vi "C-Scan (LLC messages).vi"(7 "Micropulse # In":i32, 8 "Define C-Scan Index":T1={"Index Start"=0.0, "Index Length"=260.0, "Indexing\nResolution"=5.0, "Ch1 Start"=0.0, "Ch1 Finish"=0.0, "Ch2 Start"=0.0, "Ch2 Finish"=0.0} {"Ch2 Finish" format="%#_6f"; "Ch2 Start" format="%#_6f"; "Ch1 Finish" format="%#_6f"; "Ch1 Start" format="%#_6f"; "Index Start" format="%#_6f"; "Index Length" format="%#_6f"; "Indexing\nResolution" format="%#_6f"}, 9 "Scan definition":T2={"Scan Start"=0.0, "Scan Length"=280.0, "Inspection Resolution"=0.5, "Direction"=enum."Forwards"} {"Inspection Resolution" format="%#_6f"; "Scan Start" format="%#_6f"; "Scan Length" format="%#_6f"}, 10 "Axis No.":u8=1 min=1 max=4, 11 "scan data info":T4 {"Error Message" format="%04x"; "Message Header" format="%04x"; "IP"."MIP location" format="%#.0f"; "IP"."Location" format="%#.0f"; "PRF" format="%.0fHz"}) -> (0 "Update Display?":bool, 1 "C-Scan In Progress?":bool, 2 "B-Scan index":i32, 3 "C-Scan Out":u16[][](array[numeric]))   [LabVIEW 2026, in "MicroPulse_Driver.lvlib"]
uses:
  MicroPulse_Driver.lvlib
  Data/Datatypes/MP - scan data info.ctl
  Data/Datatypes/MP - data output format.ctl
  Data/Datatypes/MP - retain scan.ctl
  Data/Datatypes/MP - axis positions (LLC).ctl
  Data/Datatypes/MP - fly scan range.ctl
  Data/Datatypes/MP - inspection direction.ctl
  Data/Datatypes/MP - C-Scan Definition.ctl
  Low Level/FGV - C-Scan Active - Action [Enum].ctl
  <instrlib>/Micropulse/Micropulse.lvlib
panel:
  out "C-Scan index":i32
  # "C-Scan Index"
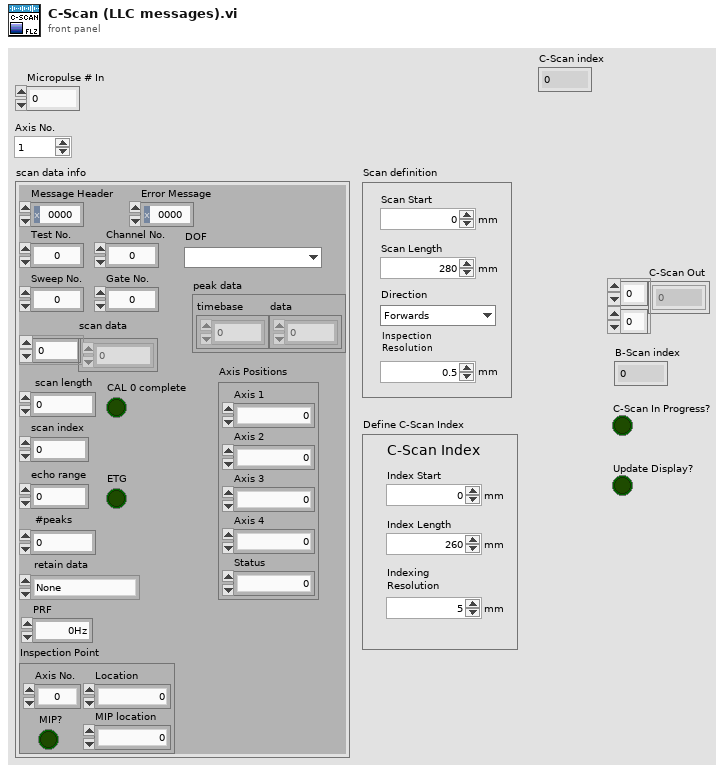
[diagram p1: front panel]
types:
  T1 = typedef "Micropulse.lvlib/MP - C-Scan Definition.ctl" = cluster{"Index Start":dbl, "Index Length":dbl, "Indexing\nResolution":dbl, "Ch1 Start":dbl, "Ch1 Finish":dbl, "Ch2 Start":dbl, "Ch2 Finish":dbl}
  T2 = typedef "Micropulse.lvlib/MP - fly scan range.ctl" = cluster{"Scan Start":dbl, "Scan Length":dbl, "Inspection Resolution":dbl, "Direction":T3}
  T3 = typedef "Micropulse.lvlib/MP - inspection direction.ctl" = enum16{"Forwards", "Backwards"}
  T4 = typedef "Micropulse.lvlib/MP - scan data info.ctl" = cluster{"Message Header":u16, "Error Message":u16, "Test No.":u32, "Channel No.":u8, "Sweep No.":u32, "Gate No.":u32, "DOF":T5, "retain data":T6, "scan data":u16[], "scan length":i32, "scan index":i32, "peak data":cluster{"timebase":u16[], "data":u16[]}, "#peaks":i32, "PRF":dbl, "IP":cluster{"Axis No.":u8, "Location":u32, "MIP location":u32, "MIP?":bool}, "echo range":u16, "ETG":bool, "CAL 0 complete":bool, "Axis Positions":T7}
  T5 = typedef "Micropulse.lvlib/MP - data output format.ctl" = enum16{"", "8-bit Mode", "10-bit Mode", "12-bit Mode", "16-bit Mode", "8-bit Log Mode", "12-bit Packed Mode"}
  T6 = typedef "Micropulse.lvlib/MP - retain scan.ctl" = enum16{"None", "Ascan", "Peaks"}
  T7 = typedef "Micropulse.lvlib/MP - axis positions (LLC).ctl" = cluster{"Axis 1":u32, "Axis 2":u32, "Axis 3":u32, "Axis 4":u32, "Status":u8}
  T8 = typedef "MicroPulse_Driver.lvlib/FGV - C-Scan Active - Action [Enum].ctl" = enum16{"Read", "Read & Reset Start Flag", "Start C-Scan", "C-Scan Finished"}
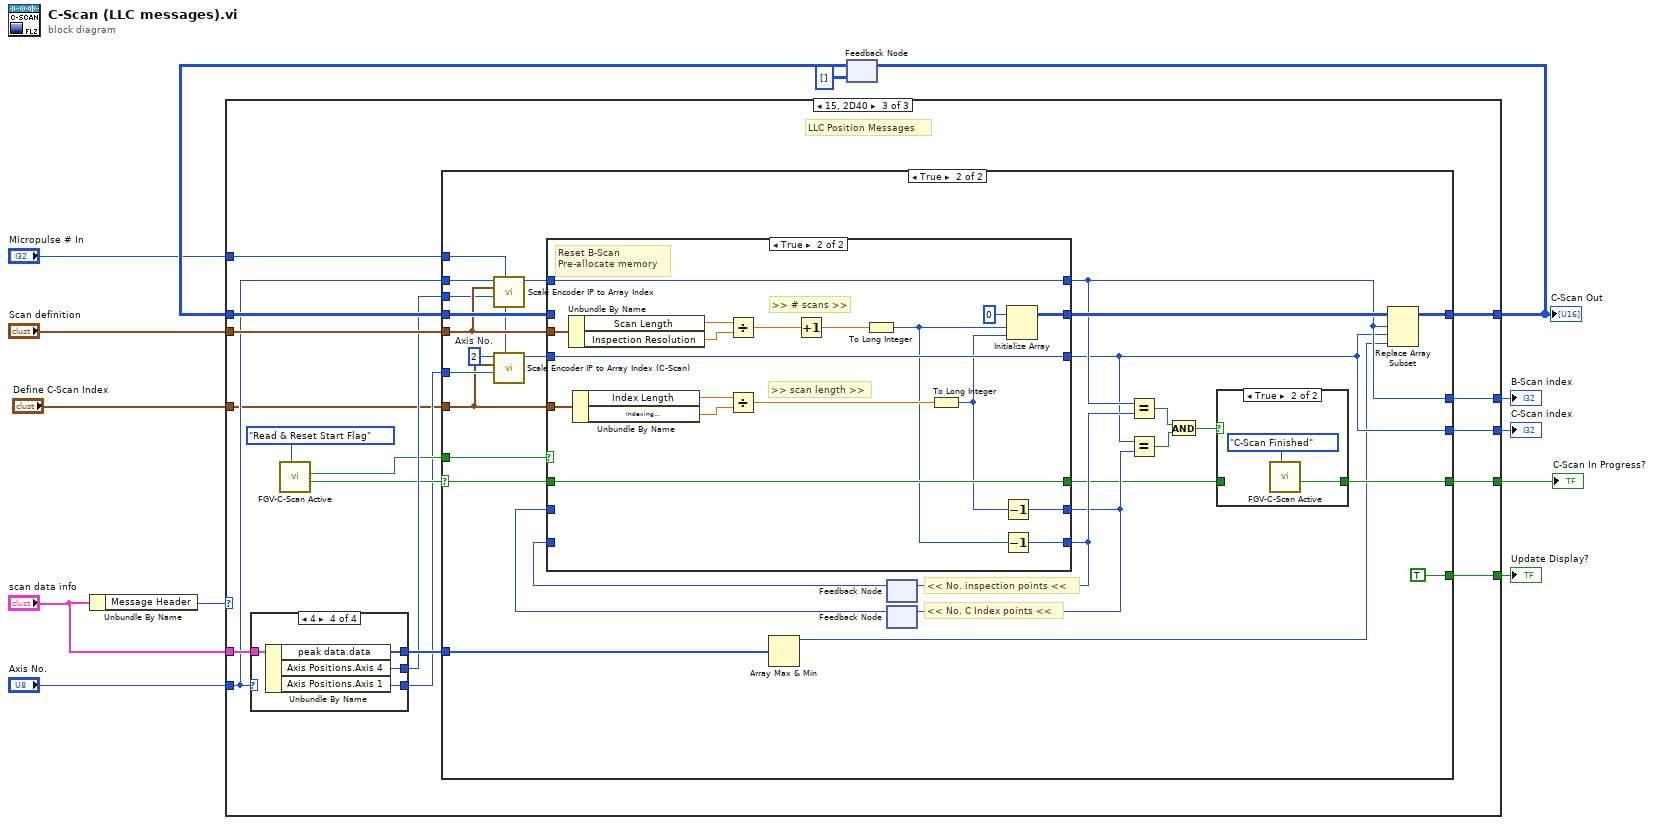
[diagram p0: block diagram]
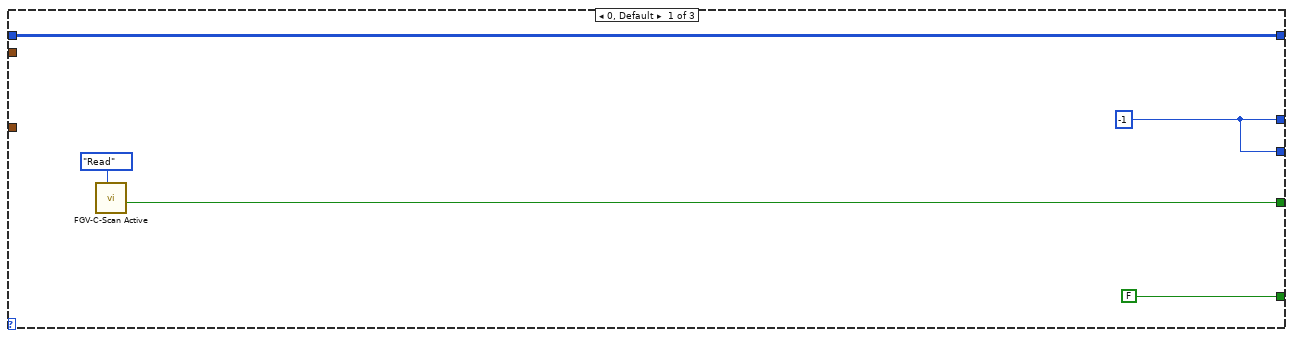
[diagram p2: hidden frame]
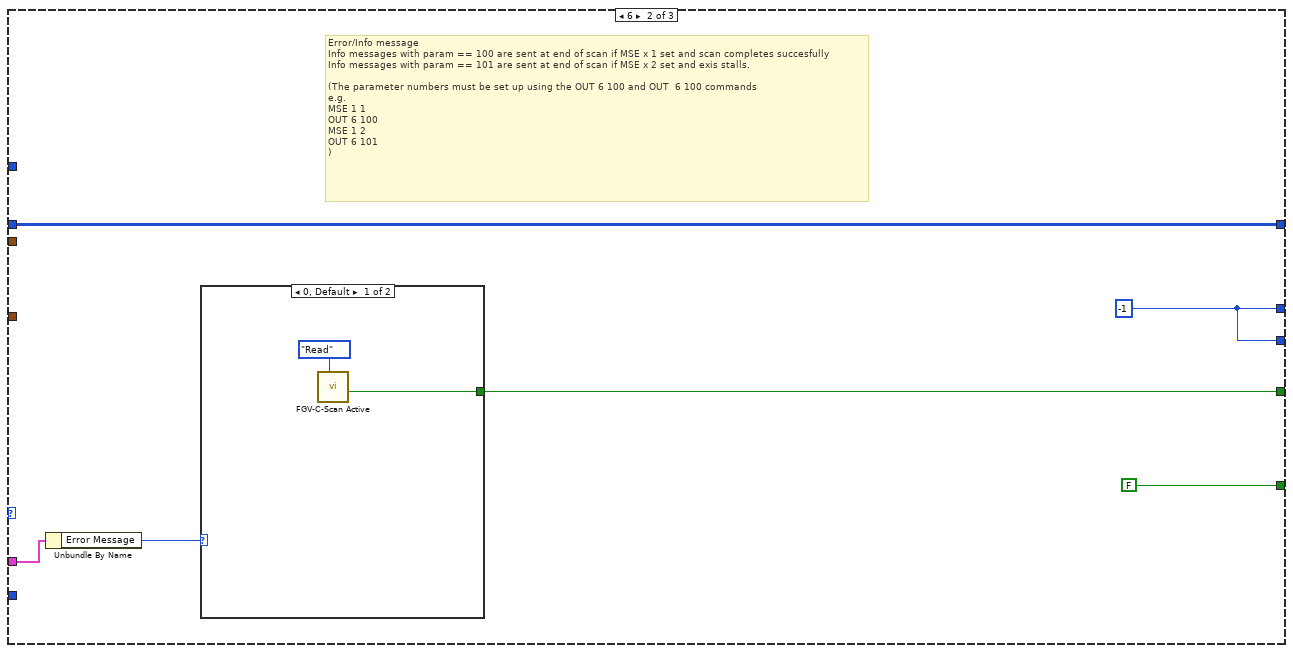
[diagram p3: hidden frame]
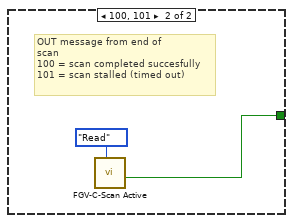
[diagram p4: hidden frame]
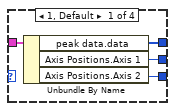
[diagram p5: hidden frame]
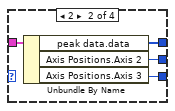
[diagram p6: hidden frame]
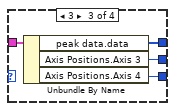
[diagram p7: hidden frame]
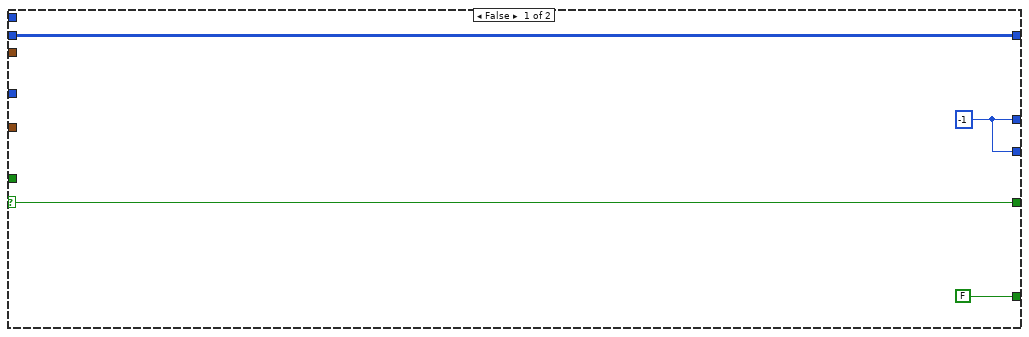
[diagram p8: hidden frame]
diagram:
  n1 = Unbundle By Name("scan data info") -> ("Message Header"=w13:u16)
  n2 = feedback #1(u16[][] []) -> (w9:u16[][])
  n3 = case shown="15, 2D40" w13 {
    tunnel: "scan data info" -> [_ w22 w45]
    tunnel: "Scan definition" -> [_ _ w39]
    tunnel: [w18 w24 w43] -> w10
    tunnel: w9 -> [w18 w24 w42]
    tunnel: "Micropulse # In" -> [_ _ w38]
    tunnel: [w14 w20 w41] -> w6
    tunnel: [FALSE FALSE w40] -> w5
    tunnel: "Axis No." -> [_ _ w36]
    tunnel: [w16 w19 w35] -> w3
    tunnel: "Define C-Scan Index" -> [_ _ w30]
    tunnel: [w16 w19 w29] -> w1
    frame 0, Default {
      w16 = -1 ("B-Scan index")
      n4 = call "FGV-C-Scan Active.vi"("Action"=FGV_-_C-Scan_Active_-_Action_[Enum]."Read") -> ("C-Scan In Progress?"=w14:bool)  [unwired: 8 in, 2 out]
    }
    frame 6 {
      w19 = -1 ("B-Scan index")
      # "Error/Info message\nInfo messages with param == 100 are sent at end of scan if MSE x 1 set and scan completes succesfully\nInfo messages with param == 101 are sent at end of scan if MSE x 2 set and exis stalls.\n\n(The parameter numbers must be set up using the OUT 6 100 and OUT  6 100 commands \ne.g.\nMSE 1 1\nOUT 6 100\nMSE 1 2\nOUT 6 101\n)"
      n5 = Unbundle By Name(w22) -> ("Error Message"=w21:u16)
      n6 = case shown="0, Default" w21 {
        tunnel: [w25 w27] -> w20
        frame 0, Default {
          n7 = call "FGV-C-Scan Active.vi"("Action"=FGV_-_C-Scan_Active_-_Action_[Enum]."Read") -> ("C-Scan In Progress?"=w25:bool)  [unwired: 8 in, 2 out]
        }
        frame 100, 101 {
          # "OUT message from end of\nscan\n100 = scan completed succesfully\n101 = scan stalled (timed out)"
          n8 = call "FGV-C-Scan Active.vi"("Action"=FGV_-_C-Scan_Active_-_Action_[Enum]."Read") -> ("C-Scan In Progress?"=w27:bool)  [unwired: 8 in, 2 out]
        }
      }
    }
    frame 21, 11584 {
      # "LLC Position Messages"
      n9 = case shown="4" w36 {
        tunnel: w45 -> [w49 w53 w57 w61]
        tunnel: [w48 w52 w56 w60] -> w44
        tunnel: [w47 w51 w55 w59] -> w37
        tunnel: [w46 w50 w54 w58] -> w31
        frame 1, Default {
          n10 = Unbundle By Name(w49) -> ("peak data.data"=w48:u16[], "Axis Positions.Axis 1"=w47:u32, "Axis Positions.Axis 2"=w46:u32)
        }
        frame 2 {
          n11 = Unbundle By Name(w53) -> ("peak data.data"=w52:u16[], "Axis Positions.Axis 2"=w51:u32, "Axis Positions.Axis 3"=w50:u32)
        }
        frame 3 {
          n12 = Unbundle By Name(w57) -> ("peak data.data"=w56:u16[], "Axis Positions.Axis 3"=w55:u32, "Axis Positions.Axis 4"=w54:u32)
        }
        frame 4 {
          n13 = Unbundle By Name(w61) -> ("peak data.data"=w60:u16[], "Axis Positions.Axis 4"=w59:u32, "Axis Positions.Axis 1"=w58:u32)
        }
      }
      n14 = call "FGV-C-Scan Active.vi"("Action"=FGV_-_C-Scan_Active_-_Action_[Enum]."Read & Reset Start Flag") -> ("C-Scan In Progress?"=w33:bool, "C-Scan Start?"=w34:bool)  [unwired: 8 in, 1 out]
      n15 = case shown="True" w33 {
        selector: w33 -> [w64 w89]
        tunnel: w42 -> [w65 w93]
        tunnel: [w65 w91] -> w43
        tunnel: w44 -> [_ w86]
        tunnel: w39 -> [_ w84]
        tunnel: [w64 w68] -> w41
        tunnel: [FALSE TRUE] -> w40
        tunnel: w38 -> [_ w67]
        tunnel: w34 -> [_ w85]
        tunnel: w37 -> [_ w83]
        tunnel: w36 -> [_ w82]
        tunnel: [w62 w76] -> w35
        tunnel: w31 -> [_ w81]
        tunnel: w30 -> [_ w79]
        tunnel: [w62 w74] -> w29
        frame False {
          w62 = -1 ("B-Scan index")
        }
        frame True {
          w80 = u8 2  # Axis No.
          # "<< No. C Index points <<"
          # "<< No. inspection points <<"
          n16 = call "Scale Encoder IP to Array Index.vi"("Micropulse # In"=w67, "Inspection Point Location"=w83, "Scan definition"=w84, "Axis No."=w82) -> ("B-Scan index"=w87:i32)  [unwired: 6 in, 1 out]
          n17 = call "Scale Encoder IP to Array Index (C-Scan).vi"("Micropulse # In"=w67, "Inspection Point Location"=w81, "Define C-Scan Index"=w79, "Axis No."=w80) -> ("C-Scan index"=w78:i32)  [unwired: 6 in, 1 out]
          n18 = Array Max & Min(array=w86) -> (max value=w66:u16)  [unwired: 3 out]
          n19 = feedback #2() -> (w90:i32)  [unwired: 1 in]
          n20 = feedback #3() -> (w77:i32)  [unwired: 1 in]
          n21 = case shown="True" w85 {
            tunnel: w93 -> [w102 _]
            tunnel: [w102 w120] -> w92
            tunnel: w84 -> [_ w118]
            tunnel: w87 -> [w100 w112]
            tunnel: [w99 w115] -> w75
            tunnel: w90 -> [w99 _]
            tunnel: [w101 w113] -> w69
            tunnel: w89 -> [w101 w113]
            tunnel: [w100 w112] -> w76
            tunnel: w79 -> [_ w109]
            tunnel: [w98 w108] -> w74
            tunnel: w78 -> [w98 w108]
            tunnel: [w97 w106] -> w73
            tunnel: w77 -> [w97 _]
            frame False {
            }
            frame True {
              # "Reset B-Scan\nPre-allocate memory"
              # ">> scan length >>"
              # ">> # scans >>"
              n22 = Unbundle By Name(w118) -> ("Scan Length"=w117:dbl, "Inspection Resolution"=w116:dbl)
              n23 = Unbundle By Name(w109) -> ("Index Length"=w110:dbl, "Indexing\nResolution"=w111:dbl)
              n24 = Divide(x=w117, y=w116) -> (x/y=w114:dbl)
              n25 = Divide(x=w110, y=w111) -> (x/y=w107:dbl)
              n26 = Increment(x=w114) -> (x+1=w103:dbl)
              n27 = To Long Integer(number=w103) -> (32bit integer=w104:i32)
              n28 = To Long Integer(number=w107) -> (32bit integer=w105:i32)
              n29 = Decrement(x=w105) -> (x-1=w106:i32)
              n30 = Decrement(x=w104) -> (x-1=w115:i32)
              n31 = Initialize Array(u16 0 ("index"), w104, w105) -> (w120:u16[][])
            }
          }
          n32 = feedback-in #2(w75) -> ()
          n33 = feedback-in #3(w73) -> ()
          n34 = Equal?(x=w76, y=w75) -> (x = y?=w72:bool)
          n35 = Equal?(x=w74, y=w73) -> (x = y?=w71:bool)
          n36 = And(x=w72, y=w71) -> (x .and. y?=w70:bool)
          n37 = case shown="True" w70 {
            tunnel: w69 -> [w94 _]
            tunnel: [w94 w95] -> w68
            frame False {
            }
            frame True {
              n38 = call "FGV-C-Scan Active.vi"("Action"=FGV_-_C-Scan_Active_-_Action_[Enum]."C-Scan Finished") -> ("C-Scan In Progress?"=w95:bool)  [unwired: 8 in, 2 out]
            }
          }
          n39 = Replace Array Subset(array=w92, new element=w66, index (row)=w76, index (col)=w74) -> (w91:u16[][])
        }
      }
    }
  }
  "C-Scan Out" <- w10
  "Update Display?" <- w5
  "C-Scan In Progress?" <- w6
  "B-Scan index" <- w3
  "C-Scan index" <- w1
  n40 = feedback-in #1(w10) -> ()
